vi "reset.vi"(3 "error in (no error)":errorcluster) -> (0 "error out":errorcluster, 1 "object list names":string[](array[string]), 2 "object list refs":refnum<class "HGF_Reference.lvclass">[](array[class]))   [LabVIEW 2012, in "HGF_ObjectManager.lvlib"]
doc: "This VI resets the internal FGV and returns object references and corresponding names."
uses:
  HGF_ObjectManager.lvlib
  HGF_BaseClasses/HGF_Reference/HGF_Reference.lvclass
  action.ctl
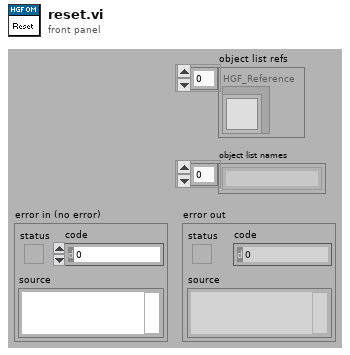
[diagram p1: front panel]
types:
  T1 = typedef "HGF_ObjectManager.lvlib/action.ctl" = enum16{"add", "remove", "name2ref", "ref2name ", "obj exists?", "cleanup", "get object list", "reset"}
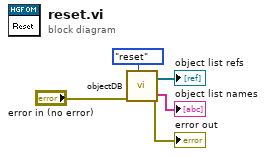
[diagram p0: block diagram]
diagram:
  n1 = call "objectDB.vi"("Action"=action."reset", "error in (no error)"="error in (no error)") -> ("error out"=→"error out":errorcluster, "object list names"=→"object list names":string[], "object list refs"=→"object list refs":refnum<class "HGF_Reference.lvclass">[])  [unwired: 3 in, 4 out]
